vi "GEA2 Stop.vi"(0 "GEA2 Reference Out":refnum<k24>, 11 "Error In":errorcluster) -> (15 "Error Out":errorcluster)   [LabVIEW 2016, in "GEA2_Toolkit.lvlib"]
doc: "This VI accepts a GEA2 bus reference and closes it. This VI should be used to close any open GEA2 connections before shutting down an application that uses the GEA2 bus."
uses:
  library/GEA2_Toolkit.lvlib
  C:/Technology Lab/NI-2010/Trunk/Utility/LabVIEW GEA2 Toolkit v1.0.0.0/Appliance.NET/GeaCommunication.dll
  Appliance.NET/GeaCommunication.dll
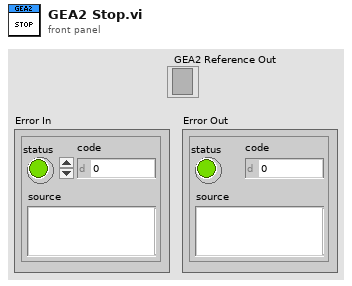
[diagram p1: front panel]
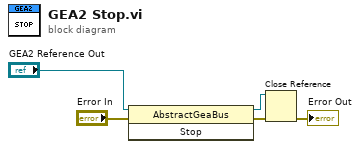
[diagram p0: block diagram]
diagram:
  n1 = invoke class="AbstractGeaBus" method="Stop"(reference="GEA2 Reference Out", error in="Error In") -> (reference out=w4:refnum<k24>, error out=w5:errorcluster)  [unwired: 1 in, 1 out]
  n2 = Close Reference(reference=w4, error in (no error)=w5) -> (error out=→"Error Out":errorcluster)
